vi "WaterValve.vi"(9 "Max pulses":u32=2) -> ()   [LabVIEW 2021]
uses:
  <vilib>/DAQmx/read.llb/DAQmx Read (Digital Bool 1Line 1Point).vi
  <vilib>/DAQmx/write.llb/DAQmx Write (Digital Bool 1Line 1Point).vi
  <vilib>/DAQmx/create/channels.llb/DAQmx Create Channel (DO-Digital Output).vi
  <vilib>/DAQmx/create/channels.llb/DAQmx Create Channel (DI-Digital Input).vi
  Global_BeamBreaks.vi
  <vilib>/DAQmx/miscellaneous.llb/DAQmx Fill In Error Info.vi
panel:
  in  "Active":bool=TRUE
  out "Number pulses":u32=51
  in  "Min IPI":u32=500
  in  "lines":tag="Dev1/port0/line1"
  in  "Open time":u32=50
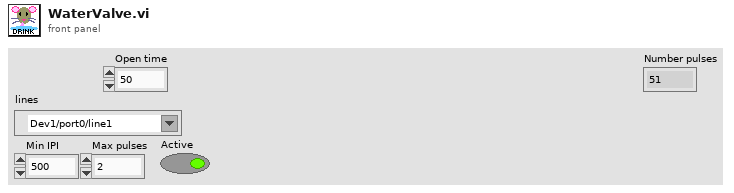
[diagram p1: front panel]
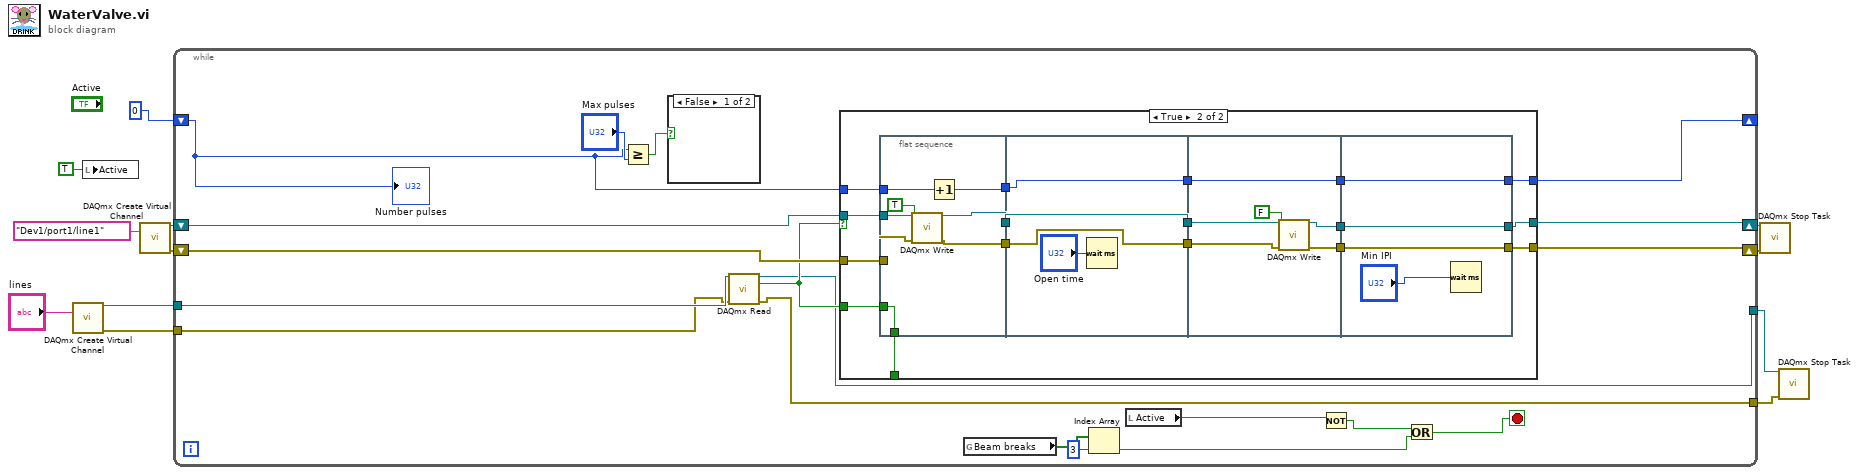
[diagram p0: block diagram]
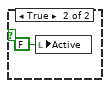
[diagram p2: hidden frame]
diagram:
  n1 = call-poly <vilib>:"DAQmx Create Virtual Channel.vi"("lines"="lines") -> ("task out"=w6:refnum<k21>, "error out"=w5:errorcluster)  [unwired: 13 in]
  n2 = local write "Active"(TRUE ("Active")) -> ()
  n3 = call-poly <vilib>:"DAQmx Create Virtual Channel.vi"("lines"=tag "Dev1/port1/line1") -> ("task out"=w11:refnum<k21>, "error out"=w10:errorcluster)  [unwired: 13 in]
  n4 = while {
    shift-right: [w29] -> w9
    shift-left: w11 -> [w31]
    shift-right: [w28] -> w8
    shift-left: w10 -> [w30]
    tunnel: w6 -> [w27]
    tunnel: w5 -> [w26]
    shift-right: [w21] -> _
    shift-left: 0 -> [w22]
    tunnel: [w19] -> w1
    tunnel: [w18] -> w2
    stop <- w13 stop-if-true
    n5 = Greater Or Equal?(x=w22, y="Max pulses") -> (x >= y?=w24:bool)
    n6 = case shown="False" w24 {
      frame False {
      }
      frame True {
        n7 = local write "Active"(FALSE ("Active")) -> ()
      }
    }
    n8 = call-poly <vilib>:"DAQmx Read.vi"("task/channels in"=w27, "error in"=w26) -> ("task out"=w19:refnum<k21>, "data"=w25:bool, "error out"=w18:errorcluster)  [unwired: 11 in]
    n9 = case shown="True" w25 {
      tunnel: w31 -> [w36 w49]
      tunnel: w30 -> [w35 w48]
      tunnel: [w36 w47] -> w29
      tunnel: [w35 w46] -> w28
      tunnel: w25 -> [w34 w45]
      tunnel: [w34 w44] -> _
      tunnel: w22 -> [w33 w40]
      tunnel: [w33 w37] -> w21
      frame False {
      }
      frame True {
        n10 = flat-sequence {
          tunnel: w49 -> [w61]
          tunnel: w48 -> [w60]
          tunnel: [w58] -> w53
          tunnel: [w57] -> w52
          tunnel: w45 -> [w56]
          tunnel: [w56] -> w44
          tunnel: [w54] -> w41
          tunnel: w40 -> [w55]
          tunnel: [w64] -> w51
          tunnel: w53 -> [w64]
          tunnel: [w63] -> w50
          tunnel: w52 -> [w63]
          tunnel: w41 -> [w62]
          tunnel: [w62] -> w38
          tunnel: w51 -> [w70]
          tunnel: w50 -> [w69]
          tunnel: [w68] -> w43
          tunnel: [w67] -> w42
          tunnel: [w66] -> w39
          tunnel: w38 -> [w66]
          tunnel: [w74] -> w46
          tunnel: [w75] -> w47
          tunnel: w43 -> [w75]
          tunnel: w42 -> [w74]
          tunnel: w39 -> [w72]
          tunnel: [w72] -> w37
          frame #0 {
            n11 = call-poly <vilib>:"DAQmx Write.vi"("task/channels in"=w61, "data"=TRUE, "error in"=w60) -> ("task out"=w58:refnum<k21>, "error out"=w57:errorcluster)  [unwired: 10 in, 1 out]
            n12 = Increment(x=w55) -> (x+1=w54:i32)
          }
          frame #1 {
            n13 = Wait (ms)(milliseconds to wait="Open time") -> ()  [unwired: 1 out]
          }
          frame #2 {
            n14 = call-poly <vilib>:"DAQmx Write.vi"("task/channels in"=w70, "data"=FALSE, "error in"=w69) -> ("task out"=w68:refnum<k21>, "error out"=w67:errorcluster)  [unwired: 10 in, 1 out]
          }
          frame #3 {
            n15 = Wait (ms)(milliseconds to wait="Min IPI") -> ()  [unwired: 1 out]
          }
        }
      }
    }
    n16 = global read "Global_BeamBreaks.vi" "Beam breaks"() -> (w17:bool[])
    n17 = Index Array(array=w17, index=3) -> (element=w14:bool)
    n18 = local read "Active"() -> (w20:bool)
    n19 = Not(x=w20) -> (.not. x?=w15:bool)
    n20 = Or(x=w15, y=w14) -> (x .or. y?=w13:bool)
    "Number pulses" <- w22
  }
  n21 = call <vilib>:"DAQmx Stop Task.vi"("task/channels in"=w9, "error in"=w8) -> ()  [unwired: 12 in, 2 out]
  n22 = call <vilib>:"DAQmx Stop Task.vi"("task/channels in"=w1, "error in"=w2) -> ()  [unwired: 12 in, 2 out]
